vi "5-Axis (Manual).vi"() -> ()   [LabVIEW 2014]
uses:
  EMC API/EMC_Typedef_Motor_Parameters.ctl
  Typedef/Typedef_Motor_Action.ctl
  Functional_Global/Typedef_FPGA_Interface_Action.ctl
  <vilib>/Motion/Express/_s/nimc.ex.clearFaults.clearFaults.axis.vi
  <vilib>/Motion/Express/_s/nimc.ex.power.power.axis.vi
  <vilib>/Motion/Express/_s/nimc.ex.resetPosition.resetPosition.axis.vi
  <vilib>/Motion/Express/_s/nimc.ex.read.readTrajectoryData.axis.vi
  <vilib>/Motion/Express/_s/nimc.ex.read.readMotionIO.axis.vi
  <vilib>/Motion/Express/_s/nimc.ex.findReferenceMove.startReferenceMove.axis.modeReverseLimit.vi
  <vilib>/Motion/Express/_s/nimc.ex.findReferenceMove.startReferenceMove.axis.modeHome.vi
  <vilib>/Motion/Express/_s/nimc.ex.findReferenceMove.startReferenceMove.axis.modeForwardLimit.vi
  <vilib>/Motion/BlockNode/FB.NIMotion.xnode
panel:
  in  "resource":refnum<k21>="Axis 1"
  out "home active":bool
  out "rev. limit active":bool
  out "fwd. limit active":bool
  out "XY Graph":cluster{"X Array":dbl[], "Y Array":dbl[]}(graph)
  in  "interval":dbl=0.01 format="%#_13g"
  in  "Gear in/out":enum16{"Gear in", "Gear out"}(ring)
  in  "denominator":i32=1
  in  "numerator":i32=1
  in  "Master Axis":T1(ring)
  out "Array":dbl[](array[knob]) scale=0.0..1000.0
  in  "Clear Errors":bool
  in  "Command":T2
  in  "Motion Parameters":T3={"position"=1000.0, "velocity"=1000.0, "acceleration"=10000.0, "deceleration"=10000.0, "accel. jerk"=10000.0, "decel. jerk"=10000.0}
  in  "Axis Index":T1(ring)
  out "error":errorcluster
  out "Numeric":i32
  in  "Stop all motors":bool
  in  "Execute Command":bool
  in  "stop":bool
  out "Axis Velocities":T4(graph)
  out "Axis Positions":T4(graph)
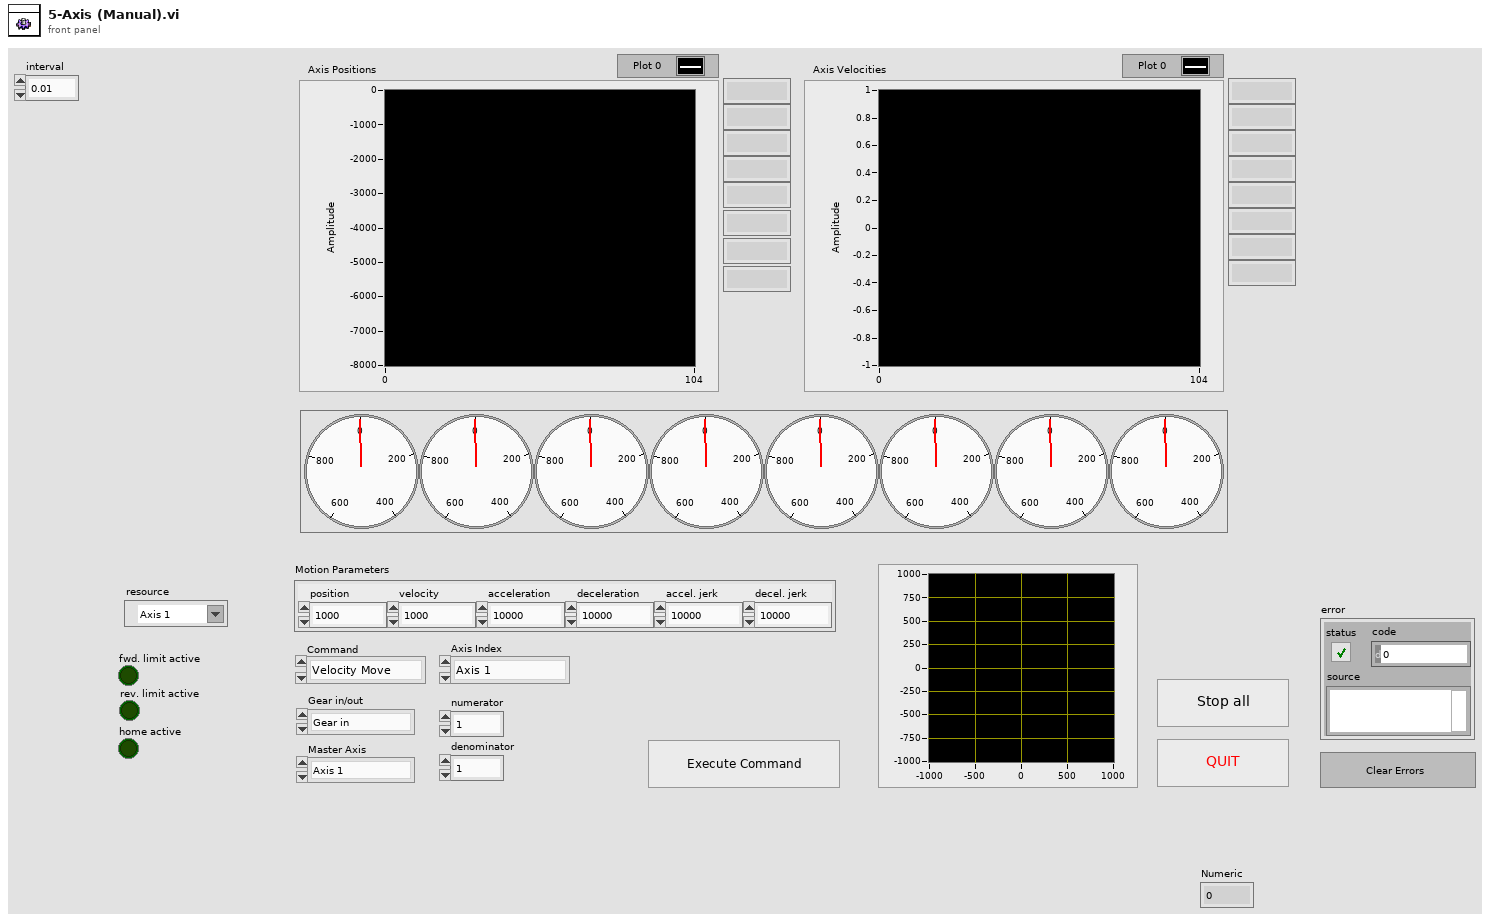
[diagram p1: front panel]
types:
  T1 = enum16{"Axis 1", "Axis 2", "Axis 3", "Axis 4", "Axis 5", "Axis 6", "Axis 7", "Axis 8"}
  T2 = typedef "Typedef_Motor_Action.ctl" = enum16{"Velocity Move", "REL Pos Move", "ABS Pos Move", "Stop", "Reset Position", "Coordinate_move", "Contour_move", "Gearing", "Find Fwd Limit", "Find Rev Limit", "Find Home"}
  T3 = typedef "EMC_Typedef_Motor_Parameters.ctl" = cluster{"position":dbl, "velocity":dbl, "acceleration":dbl, "deceleration":dbl, "accel. jerk":dbl, "decel. jerk":dbl}
  T4 = cluster{"[0]":dbl, "[1]":dbl, "[2]":dbl, "[3]":dbl, "[4]":dbl, "[5]":dbl, "[6]":dbl, "[7]":dbl}
  T5 = typedef "Typedef_FPGA_Interface_Action.ctl" = enum16{"Initialize FPGA", "Get FPGA Reference", "Close FPGA"}
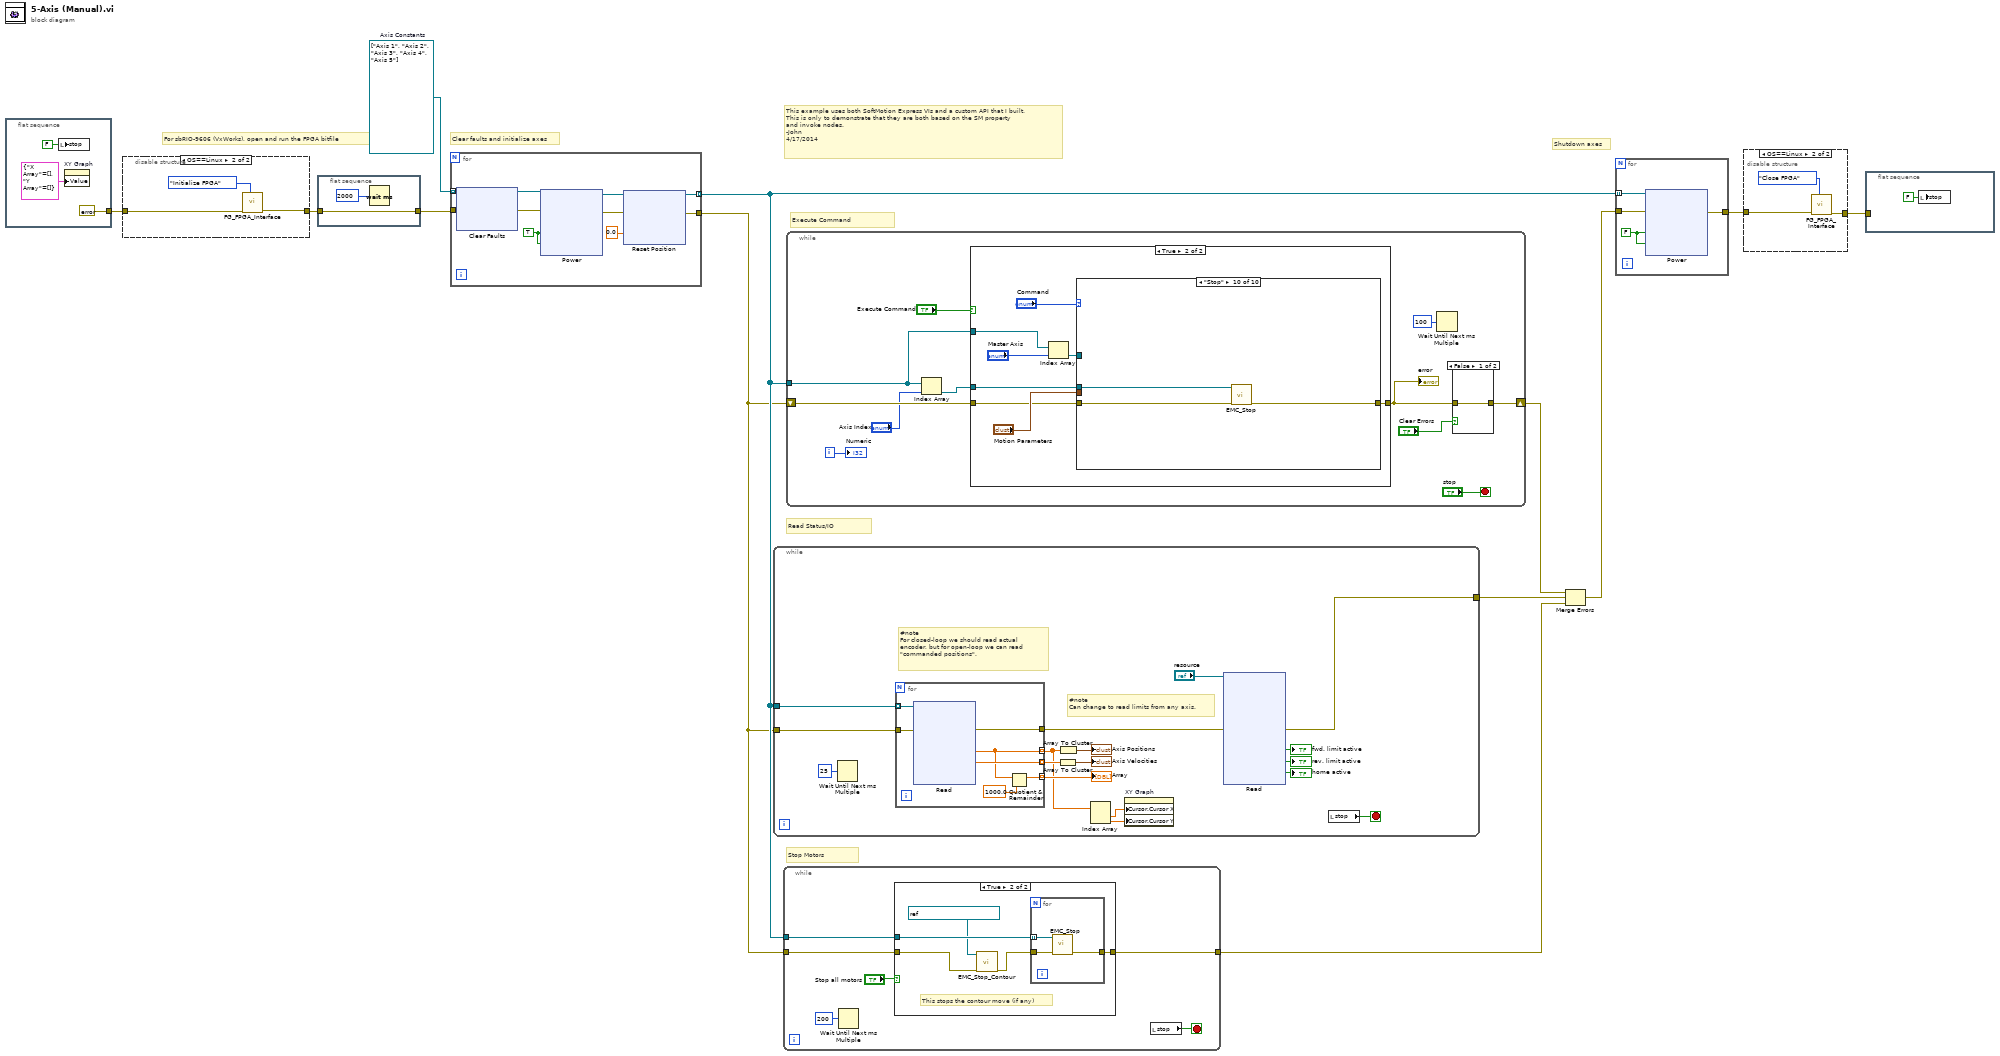
[diagram p0: block diagram]
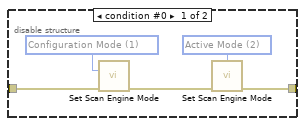
[diagram p2: hidden frame]
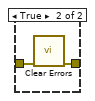
[diagram p5: hidden frame]
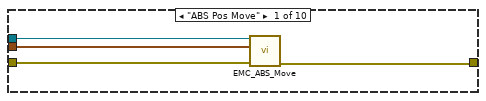
[diagram p7: hidden frame]
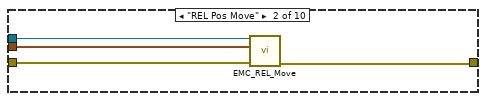
[diagram p8: hidden frame]
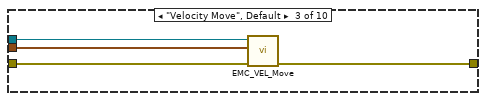
[diagram p9: hidden frame]
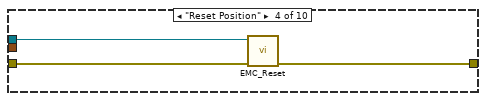
[diagram p10: hidden frame]
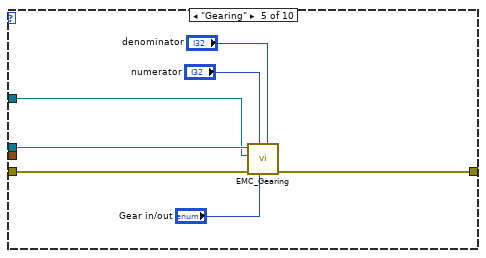
[diagram p11: hidden frame]
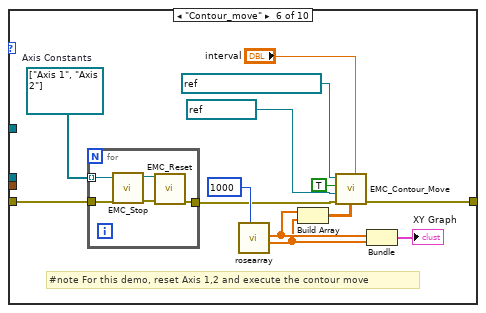
[diagram p12: hidden frame]
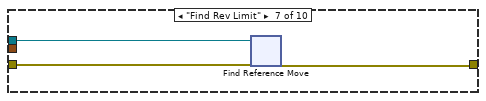
[diagram p13: hidden frame]
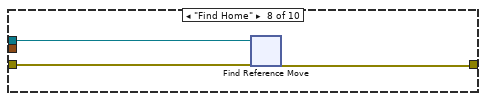
[diagram p14: hidden frame]
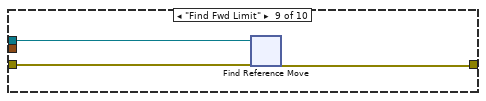
[diagram p15: hidden frame]
diagram:
  w11 = refnum<k21>[] ["Axis 1", "Axis 2", "Axis 3", "Axis 4", "Axis 5"]  # Axis Constants
  # "For sbRIO-9606 (VxWorks), open and run the FPGA bitfile"
  # "Clear faults and initialize axes"
  # "This example uses both SoftMotion Express VIs and a custom API that I built.\nThis is only to demonstrate that they are both based on the SM property\nand invoke nodes. \n-John\n4/17/2014"
  # "Shutdown axes"
  # "Execute Command"
  # "Read Status/IO"
  # "Stop Motors"
  n1 = flat-sequence {
    tunnel: [errorcluster {"status"=FALSE, "code"=0, "source"=""} ("error in (no error)")] -> w1
    frame #0 {
      n2 = local write "stop"(FALSE ("stop")) -> ()
      n3 = property on="XY Graph" class="XYGraph (strict)"("Value"=cluster{"X Array":dbl[], "Y Array":dbl[]} {"X Array"=[], "Y Array"=[]} ("XY Graph")) -> ()  [unwired: 2 in, 2 out]
    }
  }
  n4 = disable-structure shown="OS==Linux" {
    disable-tunnel: [w20 w21] -> w2
    disable-tunnel: w1 -> [w19 w22]
    frame condition #0 {
      w16 = 1 items=["Configuration Mode"=1, "Active Mode"=2] ("mode (Active Mode)")
      w17 = 2 items=["Configuration Mode"=1, "Active Mode"=2] ("mode (Active Mode)")
      n5 = call <vilib>:"Set Scan Engine Mode.vi"("mode (Active Mode)"=w16, "error in (no error)"=w19) -> ("error out"=w18:errorcluster)  [unwired: 13 in]
      n6 = call <vilib>:"Set Scan Engine Mode.vi"("mode (Active Mode)"=w17, "error in (no error)"=w18) -> ("error out"=w20:errorcluster)  [unwired: 13 in]
    }
    frame condition #1 (active) {
      n7 = call "FG_FPGA_Interface.vi"("Action"=Typedef_FPGA_Interface_Action."Initialize FPGA", "error in"=w22) -> ("error out"=w21:errorcluster)  [unwired: 8 in, 1 out]
    }
  }
  n8 = flat-sequence {
    tunnel: w2 -> [w24]
    tunnel: [w24] -> w4
    frame #0 {
      n9 = Wait (ms)(milliseconds to wait=u32 2000) -> ()  [unwired: 1 out]
    }
  }
  n10 = for {
    tunnel: w11 -> [w29] mode=indexing
    tunnel: w4 -> [w28]
    tunnel: [w31] -> w3
    tunnel: [w30] -> w5 mode=indexing
    w35 = TRUE ("enable axis")
    n11 = xnode ("Clear Faults")("resource"=w29, "error in"=w28) -> ("resource out"=w27:refnum<k21>, "error out"=w26:errorcluster)
    n12 = xnode ("Power")("enable axis"=w35, "enable drive"=w35, "resource"=w27, "error in"=w26) -> ("resource out"=w34:refnum<k21>, "error out"=w33:errorcluster)
    n13 = xnode ("Reset Position")("position"=0.0, "resource"=w34, "error in"=w33) -> ("resource out"=w30:refnum<k21>, "error out"=w31:errorcluster)
  }
  n14 = while {
    tunnel: w3 -> [w67]
    tunnel: w5 -> [w66]
    tunnel: [w55] -> w10
    stop <- w71 stop-if-true
    # "#note \nCan change to read limits from any axis."
    # "#note \nFor closed-loop we should read actual \nencoder, but for open-loop we can read\n\"commanded positions\"."
    n15 = Wait Until Next ms Multiple(millisecond multiple=u32 25) -> ()  [unwired: 1 out]
    n16 = for {
      tunnel: [w106] -> w57
      tunnel: [w101] -> w64 mode=indexing
      tunnel: [w105] -> w70 mode=indexing
      tunnel: w67 -> [w104]
      tunnel: w66 -> [w103] mode=indexing
      tunnel: [w100] -> w65 mode=indexing
      n17 = xnode ("Read")("resource"=w103, "error in"=w104) -> ("commanded position"=w101:dbl, "commanded vel."=w105:dbl, "error out"=w106:errorcluster)  [unwired: 2 out]
      n18 = Quotient & Remainder(x=w101, y=1000.0) -> (x-y*floor(x/y)=w100:dbl)  [unwired: 1 out]
    }
    "Array" <- w65
    n19 = Array To Cluster(array=w70) -> (cluster=→"Axis Velocities":T4)
    n20 = Array To Cluster(array=w64) -> (cluster=→"Axis Positions":T4)
    n21 = Index Array(array=w64) -> (element #1=w63:dbl, element #2=w62:dbl)  [unwired: 2 in]
    n22 = property on="XY Graph" class="XYGraph (strict)"("Cursor.Cursor X"=w63, "Cursor.Cursor Y"=w62) -> ()  [unwired: 2 in, 2 out]
    n23 = xnode ("Read")("resource"="resource", "error in"=w57) -> ("fwd. limit active"=→"fwd. limit active":bool, "rev. limit active"=→"rev. limit active":bool, "home active"=→"home active":bool, "error out"=w55:errorcluster)  [unwired: 6 out]
    n24 = local read "stop"() -> (w71:bool)
  }
  n25 = while {
    tunnel: w3 -> [w118]
    tunnel: w5 -> [w116]
    tunnel: [w114] -> w12
    stop <- w119 stop-if-true
    n26 = Wait Until Next ms Multiple(millisecond multiple=u32 200) -> ()  [unwired: 1 out]
    n27 = case shown="True" "Stop all motors" {
      tunnel: w118 -> [w120 w123]
      tunnel: [w120 w125] -> w114
      tunnel: w116 -> [_ w124]
      frame False {
      }
      frame True {
        # "This stops the contour move (if any)"
        n28 = call "EMC_Stop_Contour.vi"("error in (no error)"=w123, "coordinate"=refnum<k21> "Coordinate Space 1") -> ("error out"=w121:errorcluster)  [unwired: 9 in]
        n29 = for {
          tunnel: w121 -> [w128]
          tunnel: w124 -> [w126] mode=indexing
          tunnel: [w127] -> w125
          n30 = call "EMC_Stop.vi"("error in (no error)"=w128, "axis"=w126) -> ("error out"=w127:errorcluster)  [unwired: 8 in, 1 out]
        }
      }
    }
    n31 = local read "stop"() -> (w119:bool)
  }
  n32 = while {
    tunnel: w5 -> [w129]
    shift-right: [w130] -> w8
    shift-left: w3 -> [w134]
    i -> [w139]
    stop <- "stop" stop-if-true
    n33 = Index Array(array=w129, index="Axis Index") -> (element=w135:refnum<k21>)
    n34 = case shown="True" "Execute Command" {
      tunnel: w134 -> [w143 w150]
      tunnel: w135 -> [_ w149]
      tunnel: [w143 w148] -> w131
      tunnel: w129 -> [_ w145]
      frame False {
      }
      frame True {
        n35 = Index Array(array=w145, index="Master Axis") -> (element=w144:refnum<k21>)
        n36 = case shown="\"Stop\"" "Command" {
          tunnel: "Motion Parameters" -> [w152 w156 w163 _ _ _ _ _ _ _]
          tunnel: w150 -> [w155 w159 w162 w166 w173 w176 w193 w212 w233 w253]
          tunnel: w149 -> [w153 w157 w161 w165 w172 _ w192 w211 w232 w251]
          tunnel: [w154 w158 w160 w164 w171 w186 w194 w213 w234 w252] -> w148
          tunnel: w144 -> [_ _ _ _ w167 _ _ _ _ _]
          frame "ABS Pos Move" {
            n37 = call "EMC_ABS_Move.vi"("error in (no error)"=w155, "Motion Parameters"=w152, "axis"=w153) -> ("error out"=w154:errorcluster)  [unwired: 8 in]
          }
          frame "REL Pos Move" {
            n38 = call "EMC_REL_Move.vi"("error in (no error)"=w159, "Motion Parameters"=w156, "axis"=w157) -> ("error out"=w158:errorcluster)  [unwired: 8 in]
          }
          frame "Velocity Move", Default {
            n39 = call "EMC_VEL_Move.vi"("error in (no error)"=w162, "Motion Parameters"=w163, "axis"=w161) -> ("error out"=w160:errorcluster)  [unwired: 8 in]
          }
          frame "Reset Position" {
            n40 = call "EMC_Reset.vi"("error in (no error)"=w166, "axis"=w165) -> ("error out"=w164:errorcluster)  [unwired: 9 in]
          }
          frame "Gearing" {
            n41 = call "EMC_Gearing.vi"("denominator"="denominator", "Gear in/out"="Gear in/out", "numerator"="numerator", "error in (no error)"=w173, "master axis"=w167, "axis"=w172) -> ("error out"=w171:errorcluster)  [unwired: 5 in]
          }
          frame "Contour_move" {
            w174 = refnum<k21>[] ["Axis 1", "Axis 2"]  # Axis Constants
            # "#note For this demo, reset Axis 1,2 and execute the contour move"
            n42 = for {
              tunnel: w176 -> [w190]
              tunnel: [w191] -> w175
              tunnel: w174 -> [w188] mode=indexing
              n43 = call "EMC_Stop.vi"("error in (no error)"=w190, "axis"=w188) -> ("error out"=w189:errorcluster, "axis out"=w187:refnum<k21>)  [unwired: 8 in]
              n44 = call "EMC_Reset.vi"("error in (no error)"=w189, "axis"=w187) -> ("error out"=w191:errorcluster)  [unwired: 9 in]
            }
            n45 = call "rosearray.vi"("Iterations"=u32 1000) -> ("Y Array"=w178:dbl[], "X Array"=w179:dbl[])  [unwired: 5 in, 1 out]
            n46 = Build Array(w179, w178) -> (w182:dbl[][])
            n47 = call "EMC_Contour_Move.vi"("interval"="interval", "points[][]"=w182, "error in (no error)"=w175, "table"=refnum<k21> "Table 1" ("resource"), "overwrite"=TRUE, "coordinate"=refnum<k21> "Coordinate Space 1" ("resource")) -> ("error out"=w186:errorcluster)  [unwired: 5 in]
            n48 = Bundle("X Array"=w179, "Y Array"=w178) -> (→"XY Graph":cluster{"X Array":dbl[], "Y Array":dbl[]})  [unwired: 1 in]
          }
          frame "Find Rev Limit" {
            n49 = xnode "Find Reference Move"("resource"=w192, "error in"=w193) -> ("error out"=w194:errorcluster)  [unwired: 9 in, 2 out]
          }
          frame "Find Home" {
            n50 = xnode "Find Reference Move"("resource"=w211, "error in"=w212) -> ("error out"=w213:errorcluster)  [unwired: 11 in, 2 out]
          }
          frame "Find Fwd Limit" {
            n51 = xnode "Find Reference Move"("resource"=w232, "error in"=w233) -> ("error out"=w234:errorcluster)  [unwired: 9 in, 2 out]
          }
          frame "Stop" {
            n52 = call "EMC_Stop.vi"("error in (no error)"=w253, "axis"=w251) -> ("error out"=w252:errorcluster)  [unwired: 8 in, 1 out]
          }
        }
      }
    }
    "error" <- w131
    n53 = Wait Until Next ms Multiple(millisecond multiple=u32 100) -> ()  [unwired: 1 out]
    n54 = case shown="False" "Clear Errors" {
      tunnel: w131 -> [w140 w142]
      tunnel: [w140 w141] -> w130
      frame False {
      }
      frame True {
        n55 = call <vilib>:"Clear Errors.vi"("error in (no error)"=w142) -> ("error out"=w141:errorcluster)  [unwired: 5 in, 1 out]
      }
    }
    "Numeric" <- w139
  }
  n56 = Merge Errors(w8, w10, w12) -> (w7:errorcluster)
  n57 = for {
    tunnel: w5 -> [w257] mode=indexing
    tunnel: [w255] -> w6
    tunnel: w7 -> [w254]
    w256 = FALSE ("enable axis")
    n58 = xnode ("Power")("enable axis"=w256, "enable drive"=w256, "resource"=w257, "error in"=w254) -> ("error out"=w255:errorcluster)  [unwired: 1 out]
  }
  n59 = disable-structure shown="OS==Linux" {
    disable-tunnel: w6 -> [w268 w270]
    disable-tunnel: [w268 w269] -> w9
    frame condition #0 {
    }
    frame condition #1 (active) {
      n60 = call "FG_FPGA_Interface.vi"("Action"=Typedef_FPGA_Interface_Action."Close FPGA", "error in"=w270) -> ("error out"=w269:errorcluster)  [unwired: 8 in, 1 out]
    }
  }
  n61 = flat-sequence {
    tunnel: w9 -> [_]
    frame #0 {
      n62 = local write "stop"(FALSE ("stop")) -> ()
    }
  }
